vi "Pfeiffer Vacuum HLT5xx Calibration.vi"(0 "COM Port Name in":refnum<visa-resource-name>="COM1", 1 "Parameter":u16(ring) items=[" Calibration State", " Acknowledge calibrationsteps", " Leakrate external testleak vacuum", " Leakrate external testleak sniff", " Leakrate internal testleak", " Calibration factor high (read only)", " Calibration factor low (read only)", " Calibration factor counter flow (read only) "], 5 "Adress of unit":u16=1 min=1 max=999 step=1, 7 "Parameter\nread only<->describe":bool, 9 "Acknowledge\nCalibrationsteps":u16(ring)=1 items=["Cancel", "ok"], 11 "error in (no error)":errorcluster, 12 "Leakrate value in":dbl=1e-07 format="%.2e") -> (4 "response (data)":string, 8 "Calibration state out":i8(ring) items=["--", "Connect TL", "Pumping", "Measure TF high", "Massadjust", "Calibrate TF high", "Calibrate TF low", "Calibrate Counter Flow", "Remove TL", "Background TF high", "Background TF low", "Background Counter Flow", "Wait for confirmation"], 15 "error out":errorcluster)   [LabVIEW 2021]
doc: "This VI is an example of how to use the Pfeiffer Vacuum subVIs programmatically. This VI first initializes the instrument, takes measurements, then closes the instrument."
uses:
  <instrlib>/Pfeiffer Vacuum/Pfeiffer Vacuum.lvlib
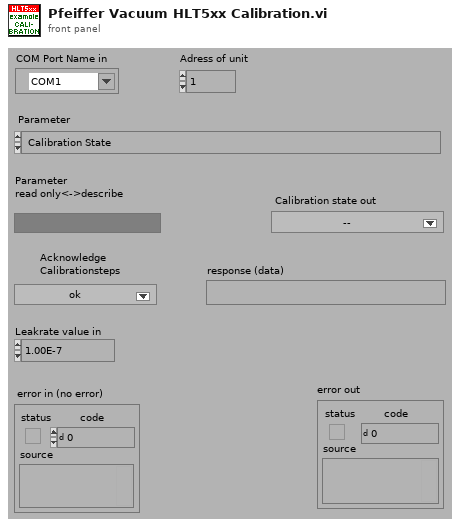
[diagram p1: front panel]
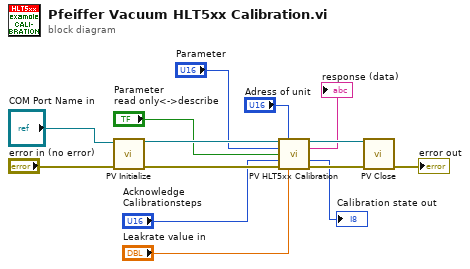
[diagram p0: block diagram]
diagram:
  n1 = call <instrlib>:"PV Initialize.vi"("error in (no error)"="error in (no error)", "VISA session in"="COM Port Name in") -> ("error out"=w14:errorcluster, "VISA session out"=w12:refnum<visa-resource-name>)  [unwired: 8 in]
  n2 = call <instrlib>:"PV HLT5xx Calibration.vi"("VISA session"=w12, "Adress of unit"="Adress of unit", "Parameter"="Parameter", "Parameter\nread only<->describe"="Parameter\nread only<->describe", "Acknowledge\nCalibrationsteps"="Acknowledge\nCalibrationsteps", "error in (no error)"=w14, "Leakrate value in"="Leakrate value in") -> ("dup VISA session"=w11:refnum<visa-resource-name>, "response (data)"=→"response (data)":string, "Calibration state out"=→"Calibration state out":i8, "error out"=w13:errorcluster)  [unwired: 5 in]
  n3 = call <instrlib>:"PV Close.vi"("VISA session"=w11, "error in (no error)"=w13) -> ("error out"=→"error out":errorcluster)  [unwired: 13 in]
